vi "Convert Radians to Degrees.vi"(1 "radians":dbl=0.700313 format="%.6f") -> (0 "degrees":dbl=40.124979238145215 format="%.3f")   [LabVIEW 2015]
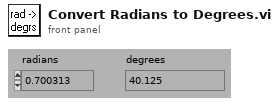
[diagram p1: front panel]
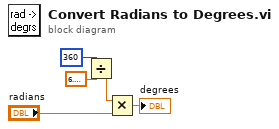
[diagram p0: block diagram]
diagram:
  n1 = Divide(x=360, y=6.283185307179586) -> (x/y=w3:dbl)
  n2 = Multiply(x=w3, y="radians") -> (x*y=→"degrees":dbl)
